vi "sendSyncMessage.vi"(8 "error in (no error)":errorcluster, 10 "interface object in":refnum<k20>, 11 "MotorControllerClass in":refnum<class "MotorControllerClass.lvclass">) -> (0 "error out":errorcluster, 2 "interface object out":refnum<k20>, 3 "MotorControllerClass out":refnum<class "MotorControllerClass.lvclass">)   [LabVIEW 2018, in "MotorControllerClass.lvclass"]
uses:
  BMS/MotorControllerClass.lvclass
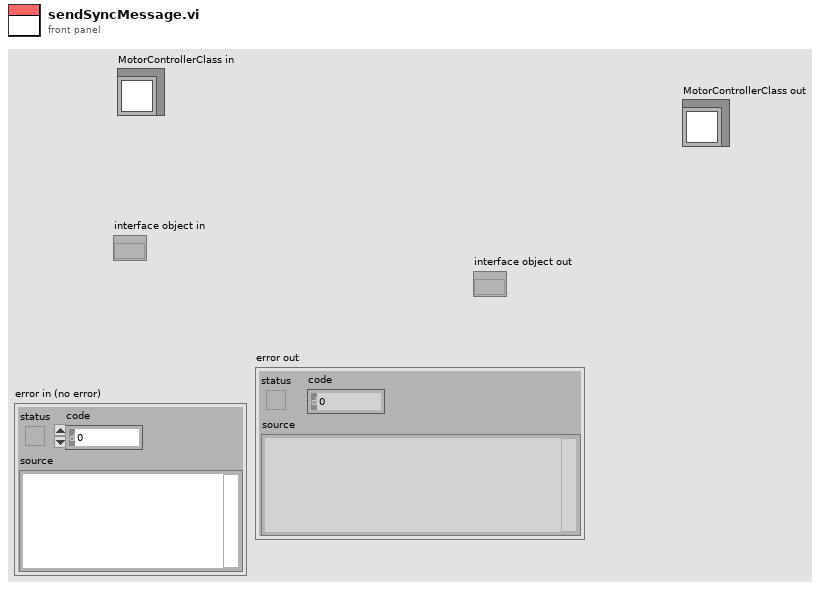
[diagram p1: front panel]
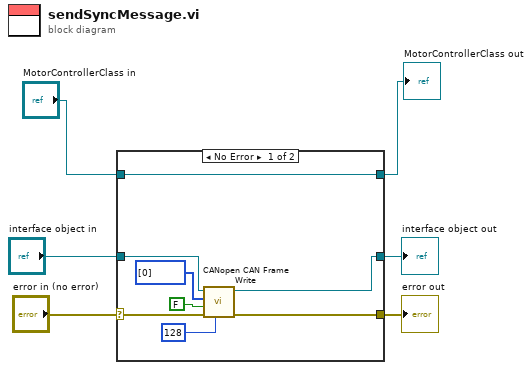
[diagram p0: block diagram]
diagram:
  n1 = case shown="No Error" "error in (no error)" {
    selector: "error in (no error)" -> [w7 w17]
    tunnel: [w11 w17] -> w5
    tunnel: [w14 w16] -> w1
    tunnel: "MotorControllerClass in" -> [w14 w16]
    tunnel: "interface object in" -> [w12 w15]
    tunnel: [w9 w15] -> w3
    frame No Error {
      n2 = call <vilib>:"CANopen CAN Frame Write.vi"("COB-ID (0)"=u32 128, "error in (no error)"=w7, "RTR? (F)"=FALSE, "CAN message data"=u8[] [0], "interface object  in"=w12) -> ("error out"=w11:errorcluster, "interface object out"=w9:refnum<k20>)  [unwired: 5 in]
    }
    frame Error {
    }
  }
  "error out" <- w5
  "interface object out" <- w3
  "MotorControllerClass out" <- w1
